vi "GetMetricDefInstance.vi"(10 "metric definition instance id":string, 11 "metric definition instances":T1[](array[typedef])) -> (1 "found":bool, 2 "metric definition instance":T1, 3 "metric definition instances out":T1[](array[typedef]))   [LabVIEW 2017, in "DeviceModelHelpers.lvlib"]
uses:
  <vilib>/addons/InsightCM/Utilities/DeviceModelHelpers/DeviceModelHelpers.lvlib
  <vilib>/addons/InsightCM/MessageBus/Base/controls/MetricDefinitionInstance.ctl
  <vilib>/addons/InsightCM/MessageBus/Base/controls/KeyValuePair.ctl
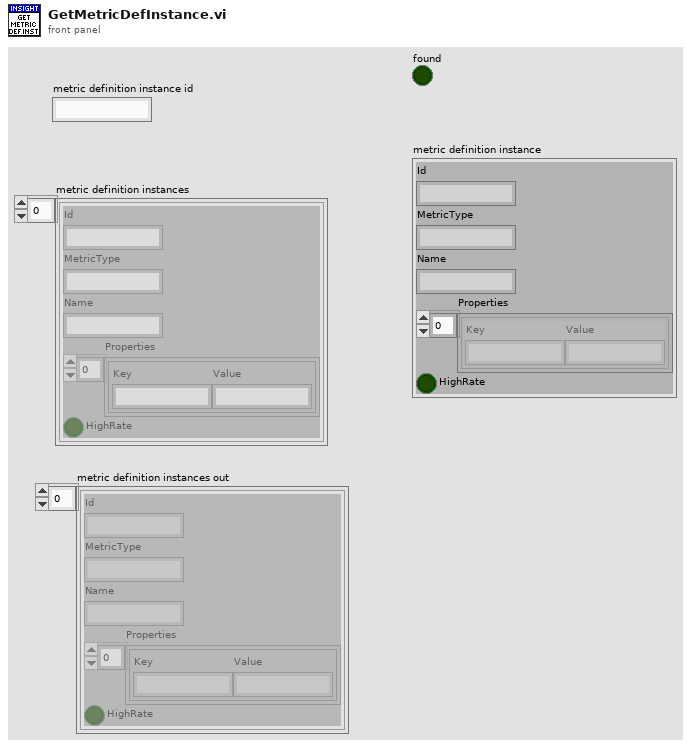
[diagram p1: front panel]
types:
  T1 = typedef "MetricDefinitionInstance.ctl" = cluster{"Id":string, "MetricType":string, "Name":string, "Properties":T2[], "HighRate":bool}
  T2 = typedef "KeyValuePair.ctl" = cluster{"Key":string, "Value":string}
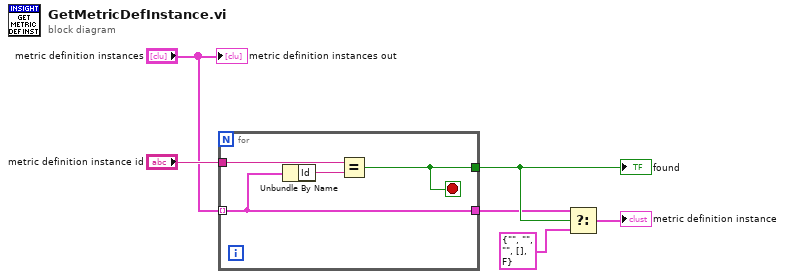
[diagram p0: block diagram]
diagram:
  n1 = for {
    tunnel: "metric definition instances" -> [w8] mode=indexing
    tunnel: "metric definition instance id" -> [w9]
    tunnel: [w8] -> w4
    tunnel: [w7] -> w5
    stop <- w7 stop-if-true
    n2 = Unbundle By Name(w8) -> ("Id"=w10:string)
    n3 = Equal?(x=w9, y=w10) -> (x = y?=w7:bool)
  }
  "found" <- w5
  n4 = Select(t=w4, s=w5, f=T1 {"Id"="", "MetricType"="", "Name"="", "Properties"=[], "HighRate"=FALSE} ("Cluster")) -> (s? t:f=→"metric definition instance":T1)
  "metric definition instances out" <- "metric definition instances"
